vi "Word Deneme.vi"() -> ()   [LabVIEW 2014]
panel:
  out "error out":errorcluster
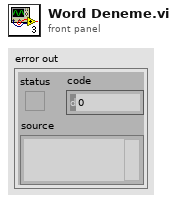
[diagram p1: front panel]
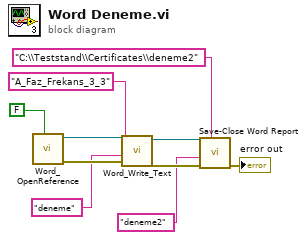
[diagram p0: block diagram]
diagram:
  n1 = call "Word_OpenReference.vi"("File Visible ?"=FALSE) -> ("error out"=w6:errorcluster, "report out"=w10:refnum<class "NI_report.lvclass">)  [unwired: 9 in]
  n2 = call "Word_Write_Text.vi"("error in (no error)"=w6, "text (\"\")"="deneme" ("text (\"\")"), "bookmark (\"\")"="A_Faz_Frekans_3_3" ("bookmark (\"\")"), "report in"=w10) -> ("error out"=w8:errorcluster, "report out"=w9:refnum<class "NI_report.lvclass">)  [unwired: 6 in]
  n3 = call "Save-Close Word Report.vi"("File Path"="C:\\Teststand\\Certificates\\deneme2", "error in (no error)"=w8, "Certificate File Name"="deneme2", "report in"=w9) -> ("error out"=→"error out":errorcluster)  [unwired: 7 in]
